vi "Time-ISO8601DueDateFixedTime.vi"(11 "Locale Time":timestamp) -> (3 "ISO 8601 Converted Due Date":string)   [LabVIEW 2014]
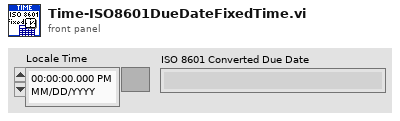
[diagram p1: front panel]
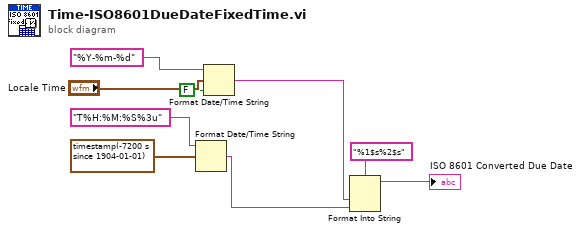
[diagram p0: block diagram]
diagram:
  n1 = Format Date/Time String(time format string (%c)="T%H:%M:%S%3u", seconds (now)=timestamp(-7200 s since 1904-01-01) ("input 1")) -> (date/time string=w8:string)  [unwired: 1 in]
  n2 = Format Date/Time String(time format string (%c)="%Y-%m-%d", seconds (now)="Locale Time", UTC format=FALSE) -> (date/time string=w7:string)
  n3 = Format Into String(format string="%1$s%2$s", w7, w8) -> (resulting string=→"ISO 8601 Converted Due Date":string)  [unwired: 2 in, 1 out]
